vi "CarSim.vi"() -> ()   [LabVIEW 2012]
uses:
  <vilib>/RTI DDS Toolkit for LabVIEW/Library/LVDDS_library.lvlib
  <vilib>/RTI DDS Toolkit for LabVIEW/VIs/Read_Num.vi
  <vilib>/RTI DDS Toolkit for LabVIEW/VIs/Write_Num.vi
  <vilib>/RTI DDS Toolkit for LabVIEW/VIs/SimpleCreateReader_NumDbl.vi
  <vilib>/RTI DDS Toolkit for LabVIEW/VIs/SimpleCreateWriter_NumDbl.vi
panel:
  out "Distance":dbl
  out "Speed":dbl(knob) scale=0.0..100.0
  out "Brake":dbl(slide) scale=0.0..100.0
  out "Gas":dbl(slide) scale=0.0..100.0
  in  "stop":bool
  in  "DomainId":u32
  # "This pane is just informative. It shows the different measures which has been\n 'Read' from the network (Gas & Brake). Also, it simulates the speed and position\na car should have, and 'Writes' these values to their corresponding topics."
  # "The DomainId should be set\nbefore run the application"
  # "Sent data"
  # "Received data"
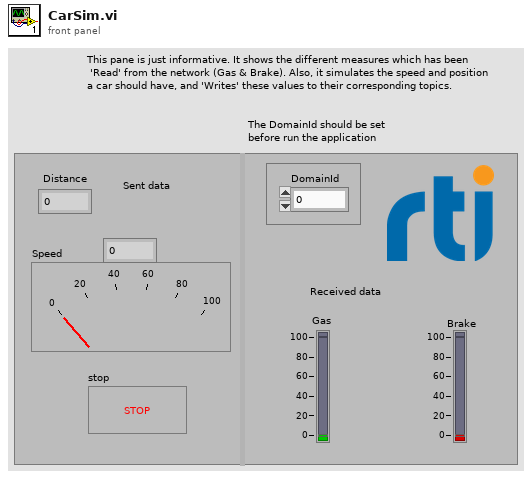
[diagram p1: front panel]
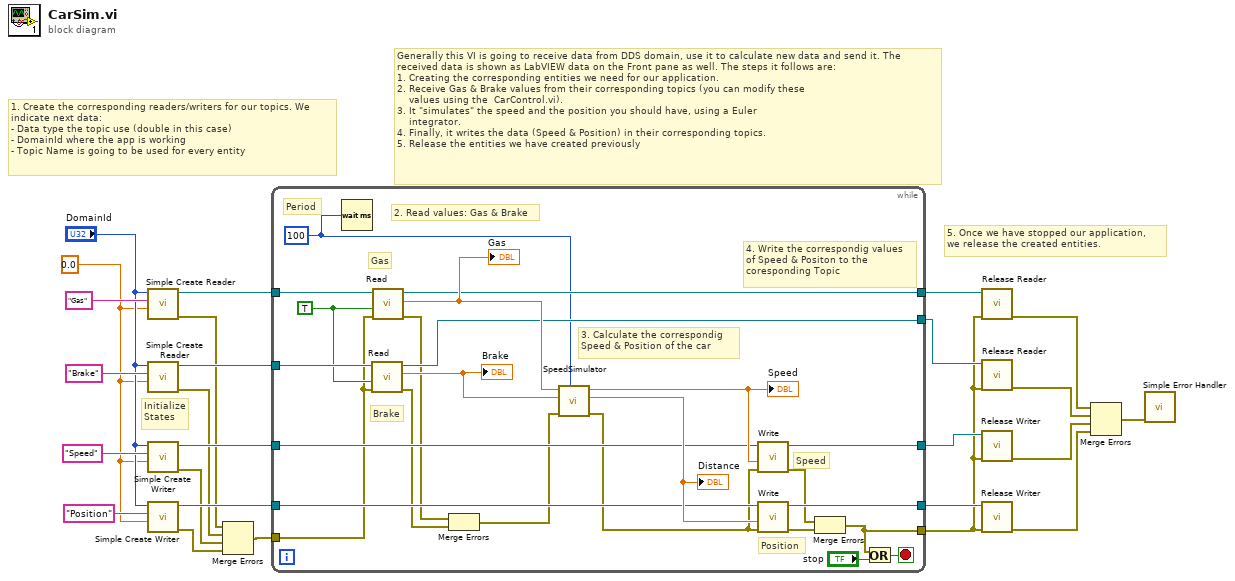
[diagram p0: block diagram]
diagram:
  w5 = 0.0
  # "5. Once we have stopped our application,\nwe release the created entities."
  # "1. Create the corresponding readers/writers for our topics. We\nindicate next data:\n- Data type the topic use (double in this case)\n- DomainId where the app is working\n- Topic Name is going to be used for every entity"
  # "Generally this VI is going to receive data from DDS domain, use it to calculate new data and send it. The\nreceived data is shown as LabVIEW data on the Front pane as well. The steps it follows are:\n1. Creating the corresponding entities we need for our application.\n2. Receive Gas & Brake values from their corresponding topics (you can modify these\n    values using the  CarControl.vi).\n3. It \"simulates\" the speed and the position you should have, using a Euler\n    integrator. \n4. Finally, it writes the data (Speed & Position) in their corresponding topics.\n5. Release the entities we have created previously"
  # "Initialize\nStates"
  n1 = call-poly <vilib>:"Simple Create Reader.vi"("data type"=w5, "topic name"="Gas", "domain id"="DomainId") -> ("error out"=w16:errorcluster, "dds read object ref"=w24:refnum<k1>)  [unwired: 7 in]
  n2 = call-poly <vilib>:"Simple Create Reader.vi"("data type"=w5, "topic name"="Brake", "domain id"="DomainId") -> ("error out"=w15:errorcluster, "dds read object ref"=w23:refnum<k1>)  [unwired: 7 in]
  n3 = call-poly <vilib>:"Simple Create Writer.vi"("data type"=w5, "topic name"="Speed", "domain id"="DomainId") -> ("error out"=w14:errorcluster, "dds writer object ref"=w21:refnum<k1>)  [unwired: 7 in]
  n4 = call-poly <vilib>:"Simple Create Writer.vi"("data type"=w5, "topic name"="Position", "domain id"="DomainId") -> ("error out"=w13:errorcluster, "dds writer object ref"=w19:refnum<k1>)  [unwired: 7 in]
  n5 = Merge Errors(w16, w15, w14, w13) -> (w12:errorcluster)
  n6 = while {
    tunnel: w24 -> [w47]
    tunnel: w21 -> [w46]
    tunnel: w23 -> [w45]
    tunnel: w19 -> [w43]
    tunnel: w12 -> [w42]
    tunnel: [w39] -> w11
    tunnel: [w38] -> w10
    tunnel: [w37] -> w4
    tunnel: [w36] -> w3
    tunnel: [w26] -> w2
    stop <- w30 stop-if-true
    w28 = u32 100 ("milliseconds to wait")
    w44 = TRUE
    # "4. Write the correspondig values\nof Speed & Positon to the \ncoresponding Topic"
    # "3. Calculate the correspondig \nSpeed & Position of the car"
    # "2. Read values: Gas & Brake"
    # "Period"
    # "Brake"
    # "Gas"
    # "Position"
    # "Speed"
    n7 = Wait (ms)(milliseconds to wait=w28) -> ()  [unwired: 1 out]
    n8 = call-poly <vilib>:"Read.vi"("error in (no error)"=w42, "only_new_samples"=w44, "dds read object ref in"=w45) -> ("error out"=w34:errorcluster, "data"=w40:dbl, "dds read object ref out"=w36:refnum<k1>)  [unwired: 5 in, 1 out]
    "Brake" <- w40
    n9 = call-poly <vilib>:"Read.vi"("error in (no error)"=w42, "only_new_samples"=w44, "dds read object ref in"=w47) -> ("error out"=w35:errorcluster, "data"=w41:dbl, "dds read object ref out"=w37:refnum<k1>)  [unwired: 5 in, 1 out]
    "Gas" <- w41
    n10 = Merge Errors(w35, w34) -> (w33:errorcluster)
    n11 = call "SpeedSimulator.vi"("Period"=w28, "error in"=w33, "Brake"=w40, "Gas"=w41) -> ("error out"=w27:errorcluster, "Distance"=w48:dbl, "Speed"=w49:dbl)  [unwired: 5 in]
    "Speed" <- w49
    "Distance" <- w48
    n12 = call-poly <vilib>:"Write.vi"("error in"=w27, "data"=w49, "dds write object ref in"=w46) -> ("error out"=w32:errorcluster, "dds write object ref out"=w39:refnum<k1>)  [unwired: 7 in]
    n13 = call-poly <vilib>:"Write.vi"("error in"=w27, "data"=w48, "dds write object ref in"=w43) -> ("error out"=w31:errorcluster, "dds write object ref out"=w38:refnum<k1>)  [unwired: 7 in]
    n14 = Merge Errors(w32, w31) -> (w26:errorcluster)
    n15 = Or(x=w26, y="stop") -> (x .or. y?=w30:bool)
  }
  n16 = call <vilib>:"Release Reader.vi"("error in"=w2, "dds read object ref in"=w4) -> ("error out"=w1:errorcluster)  [unwired: 9 in]
  n17 = call <vilib>:"Release Reader.vi"("error in"=w2, "dds read object ref in"=w3) -> ("error out"=w9:errorcluster)  [unwired: 9 in]
  n18 = call <vilib>:"Release Writer.vi"("error in"=w2, "dds write object ref"=w11) -> ("error out"=w8:errorcluster)  [unwired: 9 in]
  n19 = call <vilib>:"Release Writer.vi"("error in"=w2, "dds write object ref"=w10) -> ("error out"=w7:errorcluster)  [unwired: 9 in]
  n20 = Merge Errors(w1, w9, w8, w7) -> (w6:errorcluster)
  n21 = call <vilib>:"Simple Error Handler.vi"("error in (no error)"=w6) -> ()  [unwired: 4 in, 5 out]
